vi "Read Test Name.vi"(8 "error in (no error)":errorcluster, 11 "Null Adapter in":refnum<class "Null Adapter.lvclass">) -> (0 "error out":errorcluster, 2 "Test Name":string="Test Name", 3 "Null Adapter out":refnum<class "Null Adapter.lvclass">)   [LabVIEW 2018, in "Null Adapter.lvlib" / "Null Adapter.lvclass"]
uses:
  Null Adapter.lvclass
  Null Adapter.lvclass/Null Adapter.ctl
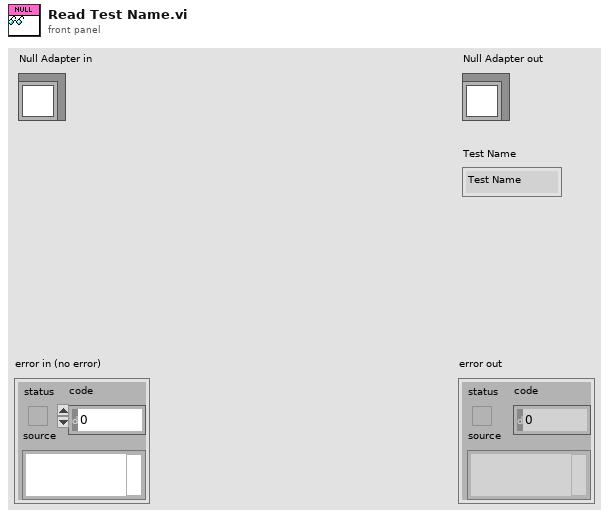
[diagram p1: front panel]
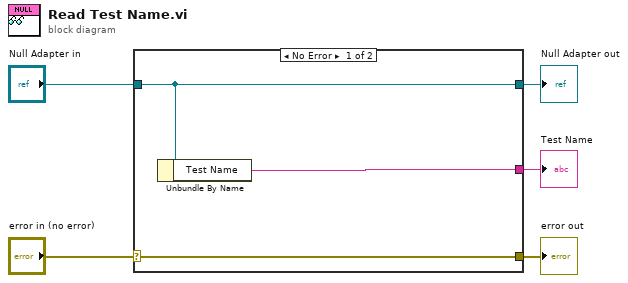
[diagram p0: block diagram]
diagram:
  n1 = case shown="No Error" "error in (no error)" {
    selector: "error in (no error)" -> [w8 w9]
    tunnel: [w8 w9] -> w4
    tunnel: [w7 w10] -> w2
    tunnel: "Null Adapter in" -> [w7 w10]
    tunnel: [w6 _] -> w1
    frame No Error {
      n2 = Unbundle By Name(w7) -> ("Test Name"=w6:string)
    }
    frame Error {
    }
  }
  "error out" <- w4
  "Null Adapter out" <- w2
  "Test Name" <- w1
